vi "PCAOM_control.vi"() -> ()   [LabVIEW 2009]
panel:
  in  "stop":bool
  in  "State":string[](array[string])=["on", "on", "on", "on", "on"]
  in  "Amplitude":string[](array[string])=["am 790", "am 720", "am 60", "am 620", "am 370"]
  in  "Frequency":string[](array[string])=["fr 52.67", "fr 57.868", "fr 62.133", "fr 66.688", "fr 74.95"]
  in  "Channel":string[](array[string])=["ch1", "ch2", "ch3", "ch4", "ch5"]
  out "error out":errorcluster
  # "MaxSetting"
  # "790"
  # "637 nm"
  # "720"
  # "594 nm"
  # "60"
  # "561 nm"
  # "620"
  # "532 nm"
  # "488 nm"
  # "370"
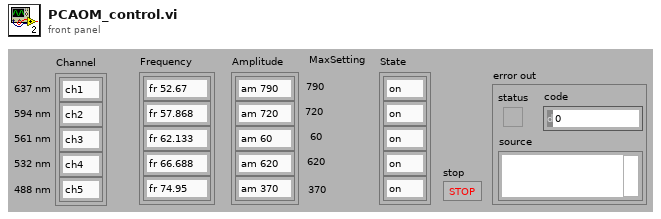
[diagram p1: front panel]
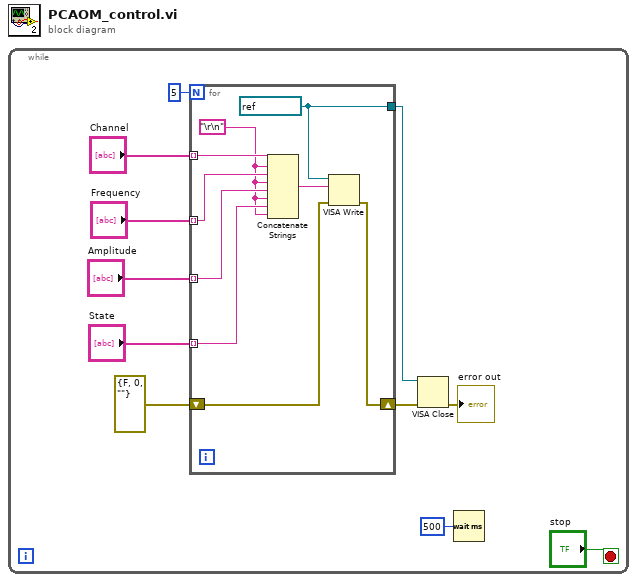
[diagram p0: block diagram]
diagram:
  n1 = while {
    stop <- "stop" stop-if-true
    n2 = for {
      N: 5 -> [_]
      tunnel: "Channel" -> [w20] mode=indexing
      tunnel: "Frequency" -> [w19] mode=indexing
      tunnel: "Amplitude" -> [w18] mode=indexing
      tunnel: "State" -> [w17] mode=indexing
      shift-right: [w13] -> w4
      shift-left: errorcluster {"status"=FALSE, "code"=0, "source"=""} ("error in (no error)") -> [w14]
      tunnel: [w12] -> w3
      w12 = refnum<visa-resource-name> "COM4" ("VISA resource name")
      w16 = "\r\n"
      n3 = Concatenate Strings(w20, w16, w19, w16, w18, w16, w17, w16) -> (w15:string)
      n4 = VISA Write(VISA resource name=w12, write buffer=w15, error in (no error)=w14) -> (error out=w13:errorcluster)  [unwired: 2 out]
    }
    n5 = VISA Close(VISA resource name=w3, error in (no error)=w4) -> (error out=→"error out":errorcluster)
    n6 = Wait (ms)(milliseconds to wait=u32 500) -> ()  [unwired: 1 out]
  }
